vi "ValveSim Main.vi"   [LabVIEW 2020, in "VolatusScratch.lvlib"]
uses:
  VolatusScratch.lvlib
  Volatus/Volatus Core/Volatus Core.lvclass
panel:
  # "ValveSim\nMain"
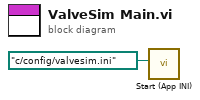
[diagram p0: block diagram]
diagram:
  n1 = call "Start (App INI).vi"("INI Path (Default)"=path "c:/config/valvesim.ini") -> ()  [unwired: 9 in, 2 out]
